vi "readConfig.vi"(8 "error in (no error)":errorcluster, 11 "Config File Name":string="config.ini") -> (0 "error out":errorcluster)   [LabVIEW 2020, in "Netatmo-WeatherStation.lvlib"]
uses:
  Netatmo-WeatherStation.lvlib
  TypeDefs/Config.ctl
  globals.vi
  <vilib>/Utility/config.llb/NI_LVConfig.lvlib
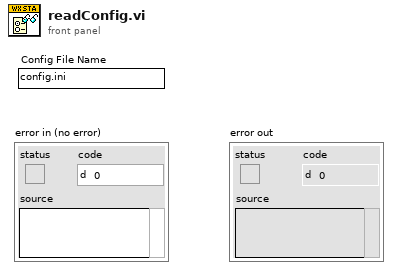
[diagram p1: front panel]
types:
  T1 = typedef "Netatmo-WeatherStation.lvlib/Config.ctl" = cluster{"Credentials":cluster{"username":string, "password":string}, "OAuth Parameters":cluster{"authorization endpoint uri":string, "token request uri":string, "grant_type":string, "scope":string}, "Client":cluster{"ID":string, "Secret":string}, "Redirect":cluster{"uri":string}, "Token":cluster{"access_token":string, "refresh_token":string, "expire_time":timestamp}}
  T2 = typedef "NI_LVConfig.lvlib/Config Data RefNum.ctl" = refnum<k1>
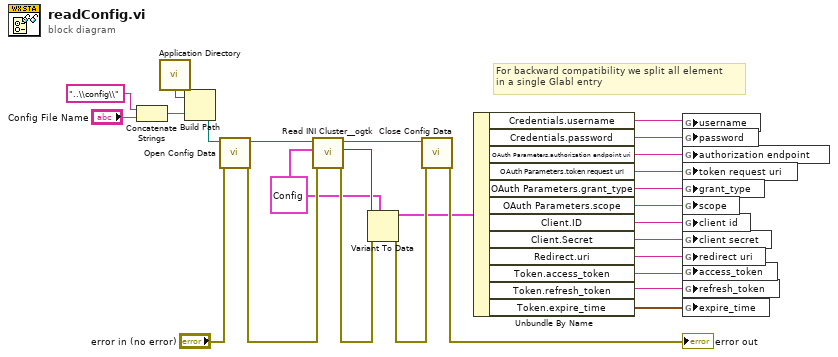
[diagram p0: block diagram]
diagram:
  w17 = T1 {"Credentials"={"username"="", "password"=""}, "OAuth Parameters"={"authorization endpoint uri"="", "token request uri"="", "grant_type"="", "scope"=""}, "Client"={"ID"="", "Secret"=""}, "Redirect"={"uri"=""}, "Token"={"access_token"="", "refresh_token"="", "expire_time"=timestamp(0 s since 1904-01-01)}} ("Config")
  # "For backward compatibility we split all element\nin a single Glabl entry"
  n1 = Concatenate Strings("..\\config\\" ("format string"), "Config File Name") -> (w3:string)
  n2 = call <vilib>:"Application Directory.vi"() -> ("Application Directory"=w25:path)
  n3 = Build Path(base path=w25, name or relative path=w3) -> (appended path=w24:path)
  n4 = call <vilib>:"Open Config Data.vi"("error in (no error)"="error in (no error)", "configuration file path"=w24) -> ("error out"=w22:errorcluster, "refnum"=w27:T2)  [unwired: 7 in, 1 out]
  n5 = call <userlib>:"Read INI Cluster__ogtk.vi"("error in (no error)"=w22, "INI Fomatted Cluster Type"=w17, "refnum"=w27) -> ("error out"=w21:errorcluster, "INI Fomatted Cluster"=w26:variant, "dup refnum"=w23:T2)  [unwired: 4 in, 2 out]
  n6 = Variant To Data(error in=w21, type=w17, Variant=w26) -> (data=w16:T1, error out=w20:errorcluster)
  n7 = call <vilib>:"Close Config Data.vi"("error in (no error)"=w20, "refnum"=w23) -> ("error out"=→"error out":errorcluster)  [unwired: 8 in, 1 out]
  n8 = Unbundle By Name(w16) -> ("Credentials.username"=w15:string, "Credentials.password"=w14:string, "OAuth Parameters.authorization endpoint uri"=w13:string, "OAuth Parameters.token request uri"=w12:string, "OAuth Parameters.grant_type"=w11:string, "OAuth Parameters.scope"=w10:string, "Client.ID"=w9:string, "Client.Secret"=w8:string, "Redirect.uri"=w7:string, "Token.access_token"=w6:string, "Token.refresh_token"=w5:string, "Token.expire_time"=w4:timestamp)
  n9 = global write "globals.vi" "username"(w15) -> ()
  n10 = global write "globals.vi" "password"(w14) -> ()
  n11 = global write "globals.vi" "authorization endpoint"(w13) -> ()
  n12 = global write "globals.vi" "token request uri"(w12) -> ()
  n13 = global write "globals.vi" "grant_type"(w11) -> ()
  n14 = global write "globals.vi" "scope"(w10) -> ()
  n15 = global write "globals.vi" "client id"(w9) -> ()
  n16 = global write "globals.vi" "client secret"(w8) -> ()
  n17 = global write "globals.vi" "redirect uri"(w7) -> ()
  n18 = global write "globals.vi" "access_token"(w6) -> ()
  n19 = global write "globals.vi" "refresh_token"(w5) -> ()
  n20 = global write "globals.vi" "expire_time"(w4) -> ()
